vi "OK.vi"(8 "error in (no error)":errorcluster, 11 "NPad2 in":refnum<class "NPad2.lvclass">) -> (0 "error out":errorcluster, 3 "NPad2 out":refnum<class "NPad2.lvclass">)   [LabVIEW 2020, in "NPad2.lvlib" / "NPad2.lvclass"]
uses:
  NPad2.lvclass
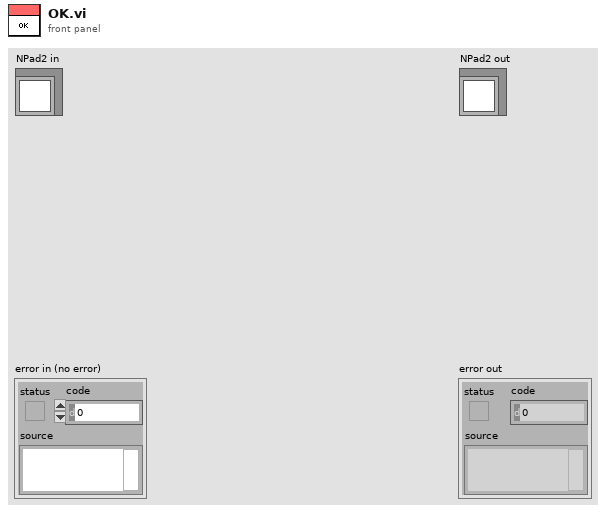
[diagram p1: front panel]
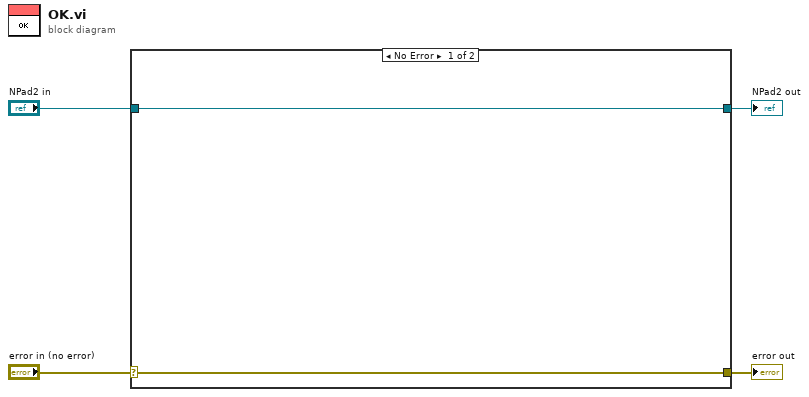
[diagram p0: block diagram]
diagram:
  n1 = case shown="No Error" "error in (no error)" {
    selector: "error in (no error)" -> [w5 w8]
    tunnel: [w5 w8] -> w3
    tunnel: [w6 w7] -> w1
    tunnel: "NPad2 in" -> [w6 w7]
    frame No Error {
    }
    frame Error {
    }
  }
  "error out" <- w3
  "NPad2 out" <- w1
